vi "Begin.vi"(8 "error in":errorcluster) -> (0 "error out":errorcluster)   [LabVIEW 2018]
doc: "Called before other user functions, this VI can be used to open I/O refnums, load in file data, and do general program initialization. Notice that the <B>error out</B> terminal is simply used for data flow. Wiring it to other structures or subVIs ensures that this VI runs first."
uses:
  <vilib>/Rock Robotics/WPI/DriverStation/WPI_DriverStationRobotMode2.ctl
  <vilib>/Rock Robotics/WPI/Joystick/WPI_JoystickDeviceEnum.ctl
  <vilib>/Rock Robotics/WPI/SafetyOutput/WPI_SafetyOutputConfigMenu.ctl
  <vilib>/Rock Robotics/WPI/Solenoid/WPI_SolenoidChannel.ctl
  <vilib>/Rock Robotics/WPI/Solenoid/WPI_SolenoidValue.ctl
  <vilib>/Rock Robotics/SystemInterfaces/DIO/FPGA_DIOPWMChannel.ctl
  Robot Global Data.vi
  <vilib>/Rock Robotics/WPI/RobotDrive/WPI_RobotDriveOpen4MotorWithExistingMotors.vi
  <vilib>/Rock Robotics/WPI/RobotDrive/WPI_RobotDriveOpen2MotorWithExistingMotors.vi
  <vilib>/Rock Robotics/WPI/Solenoid/WPI_SolenoidOpenDouble.vi
  <vilib>/Rock Robotics/WPI/Solenoid/WPI_SolenoidSetEnum.vi
  <vilib>/Rock Robotics/WPI/MotorControl/WPI_MotorControlOpen SPARK.vi
panel:
  in  "Power Distribution Panel (0)":u8
  in  "Clear Sticky Faults":bool=TRUE
  out "Current Faults":bool[](array[boolean])
  out "Battery Voltage Fault":bool
  out "Temperature Fault":bool
  out "Hardware Fault":bool
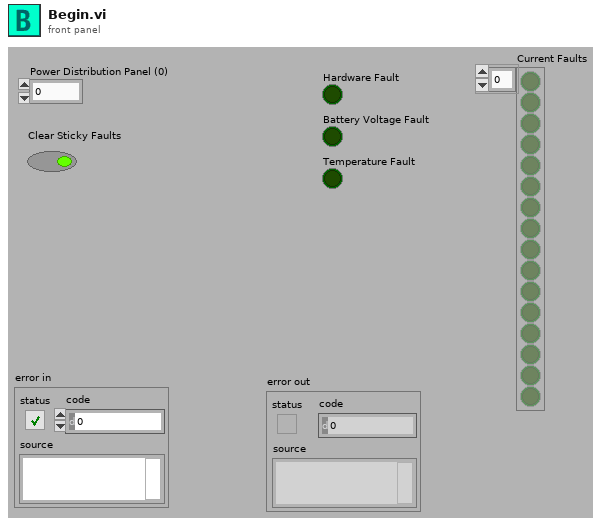
[diagram p1: front panel]
types:
  T1 = typedef "FPGA_DIOPWMChannel.ctl" = enum8{"PWM 0", "PWM 1", "PWM 2", "PWM 3", "PWM 4", "PWM 5", "PWM 6", "PWM 7", "PWM 8", "PWM 9", "PWM MXP 0", "PWM MXP 1", "PWM MXP 2", "PWM MXP 3", "PWM MXP 4", "PWM MXP 5", "PWM MXP 6", "PWM MXP 7", "PWM MXP 8", "PWM MXP 9", "Invalid"}
  T2 = typedef "WPI_SafetyOutputConfigMenu.ctl" = enum16{"Enable", "Disable"}
  T3 = typedef "WPI_SolenoidValue.ctl" = enum16{"Off", "On", "Forward", "Reverse"}
  T4 = typedef "WPI_SolenoidChannel.ctl" = enum8{"Solenoid 0", "Solenoid 1", "Solenoid 2", "Solenoid 3", "Solenoid 4", "Solenoid 5", "Solenoid 6", "Solenoid 7", "Invalid"}
  T5 = typedef "WPI_JoystickDeviceEnum.ctl" = enum16{"USB 0", "USB 1", "USB 2", "USB 3", "USB 4", "USB 5"}
  T6 = typedef "WPI_DriverStationRobotMode2.ctl" = enum16{"Autonomous Disabled", "Autonomous Enabled", "Teleop Disabled", "Teleop Enabled", "Disconnected", "Finish", "Test Disabled", "Test Enabled", "Emergency Stopped"}
  T7 = typedef "WPI_SolenoidDevRef.ctl" = cluster{"DevStatus":errorcluster, "Pneumatics Control Module":u8, "Forward Solenoid Channel":T4, "Reverse Solenoid Channel":T4}
  T8 = typedef "WPI_JoystickDevRef.ctl" = cluster{"Device":T5}
  T9 = typedef "WPI_MotorControlDeviceRef.ctl" = cluster{"DeviceStatus":errorcluster, "Type":T10, "PWM":cluster{"PWM Channel":T1, "DeadBand":T11}, "CAN":cluster{"Device Number":u8, "SetOutput VI Ref":variant, "GetOutput VI Ref":variant, "Enable VI Ref":variant, "Disable VI Ref":variant, "Data":variant}, "Invert":bool, "DIO PWM":cluster{"PWM \"Enable\" Channel":T1, "DIOChannel":T12, "PWM Rate":dbl}}
  T10 = typedef "WPI_MotorControlType.ctl" = enum16{"PWM", "CAN", "DIO PWM"}
  T11 = typedef "WPI_PWMDeadband.ctl" = cluster{"Name":string, "maxPositivePwm":i32, "minPositivePwm":i32, "centerPwm":i32, "maxNegativePwm":i32, "minNegativePwm":i32, "angularRange":u16}
  T12 = typedef "FPGA_DIOChannel.ctl" = enum8{"DIO 0", "DIO 1", "DIO 2", "DIO 3", "DIO 4", "DIO 5", "DIO 6", "DIO 7", "DIO 8", "DIO 9", "DIO MXP 0", "DIO MXP 1", "DIO MXP 2", "DIO MXP 3", "DIO MXP 4", "DIO MXP 5", "DIO MXP 6", "DIO MXP 7", "DIO MXP 8", "DIO MXP 9", "DIO MXP 10", "DIO MXP 11", "DIO MXP 12", "DIO MXP 13", "DIO MXP 14", "DIO MXP 15", "SPI Port CS1", "SPI Port CS2", "SPI Port CS3", "SPI Port MISO", "SPI Port MOSI", "Invalid"}
  T13 = typedef "WPI_RobotDriveDevRef.ctl" = cluster{"DevStatus":errorcluster, "Motors[]":T9[], "Square Inputs":bool, "Max Output":dbl}
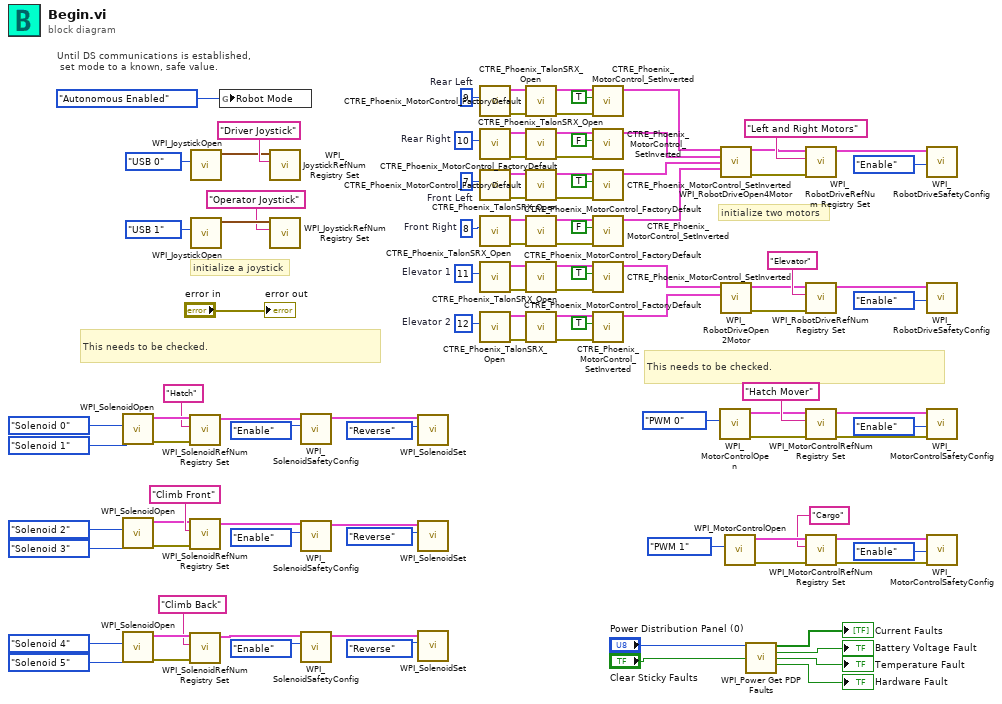
[diagram p0: block diagram]
diagram:
  w71 = u8 11  # Elevator 1
  w64 = u8 12  # Elevator 2
  w38 = u8 8  # Front Right
  w39 = u8 7  # Front Left
  w37 = u8 10  # Rear Right
  w36 = u8 9  # Rear Left
  # "This needs to be checked."
  # "This needs to be checked."
  # "initialize two motors"
  # "initialize a joystick"
  # "Until DS communications is established,\n set mode to a known, safe value."
  n1 = call-poly <vilib>:"WPI_SolenoidOpen.vi"("Reverse Solenoid Channel"=WPI_SolenoidChannel."Solenoid 1", "Forward Solenoid Channel"=WPI_SolenoidChannel."Solenoid 0" ("Solenoid Channel")) -> ("error out"=w3:errorcluster, "SolenoidDevRef"=w94:T7)  [unwired: 8 in]
  n2 = call-poly <vilib>:"WPI_SolenoidOpen.vi"("Reverse Solenoid Channel"=WPI_SolenoidChannel."Solenoid 3", "Forward Solenoid Channel"=WPI_SolenoidChannel."Solenoid 2" ("Solenoid Channel")) -> ("error out"=w2:errorcluster, "SolenoidDevRef"=w91:T7)  [unwired: 8 in]
  n3 = call-poly <vilib>:"WPI_SolenoidOpen.vi"("Reverse Solenoid Channel"=WPI_SolenoidChannel."Solenoid 5", "Forward Solenoid Channel"=WPI_SolenoidChannel."Solenoid 4" ("Solenoid Channel")) -> ("error out"=w1:errorcluster, "SolenoidDevRef"=w23:T7)  [unwired: 8 in]
  n4 = call <vilib>:"WPI_SolenoidRefNum Registry Set.vi"("error in (no error)"=w3, "refnum name"="Hatch", "SolenoidDevRef"=w94) -> ("SolenoidDevRef"=w16:T7)  [unwired: 7 in, 1 out]
  n5 = call <vilib>:"WPI_SolenoidRefNum Registry Set.vi"("error in (no error)"=w2, "refnum name"="Climb Front", "SolenoidDevRef"=w91) -> ("SolenoidDevRef"=w14:T7)  [unwired: 7 in, 1 out]
  n6 = call <vilib>:"WPI_SolenoidRefNum Registry Set.vi"("error in (no error)"=w1, "refnum name"="Climb Back", "SolenoidDevRef"=w23) -> ("SolenoidDevRef"=w12:T7)  [unwired: 7 in, 1 out]
  n7 = call <vilib>:"WPI_JoystickOpen.vi"("JoystickDevice"=WPI_JoystickDeviceEnum."USB 0") -> ("JoystickDevRef"=w29:T8)  [unwired: 10 in]
  n8 = call <vilib>:"WPI_JoystickOpen.vi"("JoystickDevice"=WPI_JoystickDeviceEnum."USB 1") -> ("JoystickDevRef"=w26:T8)  [unwired: 10 in]
  n9 = global write "Robot Global Data.vi" "Robot Mode"(WPI_DriverStationRobotMode2."Autonomous Enabled" ("Robot Mode")) -> ()
  n10 = call <vilib>:"WPI_JoystickRefNum Registry Set.vi"("refnum name"="Driver Joystick", "JoystickDevRef"=w29) -> ()  [unwired: 8 in, 2 out]
  n11 = call <vilib>:"WPI_JoystickRefNum Registry Set.vi"("refnum name"="Operator Joystick", "JoystickDevRef"=w26) -> ()  [unwired: 8 in, 2 out]
  n12 = call <vilib>:"WPI_SolenoidSafetyConfig.vi"("mode"=WPI_SafetyOutputConfigMenu."Enable", "SolenoidDevRef"=w16) -> ("SolenoidDevRef"=w15:T7)  [unwired: 8 in, 1 out]
  n13 = call <vilib>:"WPI_SolenoidSafetyConfig.vi"("mode"=WPI_SafetyOutputConfigMenu."Enable", "SolenoidDevRef"=w14) -> ("SolenoidDevRef"=w13:T7)  [unwired: 8 in, 1 out]
  n14 = call <vilib>:"WPI_SolenoidSafetyConfig.vi"("mode"=WPI_SafetyOutputConfigMenu."Enable", "SolenoidDevRef"=w12) -> ("SolenoidDevRef"=w11:T7)  [unwired: 8 in, 1 out]
  n15 = call-poly <vilib>:"WPI_SolenoidSet.vi"("Value"=WPI_SolenoidValue."Reverse", "SolenoidDevRef"=w15) -> ()  [unwired: 8 in, 2 out]
  n16 = call-poly <vilib>:"WPI_SolenoidSet.vi"("Value"=WPI_SolenoidValue."Reverse", "SolenoidDevRef"=w13) -> ()  [unwired: 8 in, 2 out]
  n17 = call-poly <vilib>:"WPI_SolenoidSet.vi"("Value"=WPI_SolenoidValue."Reverse", "SolenoidDevRef"=w11) -> ()  [unwired: 8 in, 2 out]
  n18 = call <vilib>:"CTRE_Phoenix_TalonSRX_Open.vi"("Device Number"=w36) -> ("error out"=w48:errorcluster, "CAN Talon SRX Ref"=w49:T9)  [unwired: 9 in]
  n19 = call <vilib>:"CTRE_Phoenix_TalonSRX_Open.vi"("Device Number"=w37) -> ("error out"=w50:errorcluster, "CAN Talon SRX Ref"=w51:T9)  [unwired: 9 in]
  n20 = call <vilib>:"CTRE_Phoenix_TalonSRX_Open.vi"("Device Number"=w39) -> ("error out"=w52:errorcluster, "CAN Talon SRX Ref"=w53:T9)  [unwired: 9 in]
  n21 = call <vilib>:"CTRE_Phoenix_TalonSRX_Open.vi"("Device Number"=w38) -> ("error out"=w54:errorcluster, "CAN Talon SRX Ref"=w55:T9)  [unwired: 9 in]
  n22 = call <vilib>:"CTRE_Phoenix_TalonSRX_Open.vi"("Device Number"=w71) -> ("error out"=w7:errorcluster, "CAN Talon SRX Ref"=w69:T9)  [unwired: 9 in]
  n23 = call <vilib>:"CTRE_Phoenix_TalonSRX_Open.vi"("Device Number"=w64) -> ("error out"=w5:errorcluster, "CAN Talon SRX Ref"=w66:T9)  [unwired: 9 in]
  n24 = call <vilib>:"CTRE_Phoenix_MotorControl_FactoryDefault.vi"("error in"=w48, "PhoenixMotorControlDevRef"=w49) -> ("error out"=w57:errorcluster, "PhoenixMotorControlDevRef"=w56:T9)  [unwired: 8 in]
  n25 = call <vilib>:"CTRE_Phoenix_MotorControl_FactoryDefault.vi"("error in"=w50, "PhoenixMotorControlDevRef"=w51) -> ("error out"=w59:errorcluster, "PhoenixMotorControlDevRef"=w58:T9)  [unwired: 8 in]
  n26 = call <vilib>:"CTRE_Phoenix_MotorControl_FactoryDefault.vi"("error in"=w52, "PhoenixMotorControlDevRef"=w53) -> ("error out"=w61:errorcluster, "PhoenixMotorControlDevRef"=w60:T9)  [unwired: 8 in]
  n27 = call <vilib>:"CTRE_Phoenix_MotorControl_FactoryDefault.vi"("error in"=w54, "PhoenixMotorControlDevRef"=w55) -> ("error out"=w63:errorcluster, "PhoenixMotorControlDevRef"=w62:T9)  [unwired: 8 in]
  n28 = call <vilib>:"CTRE_Phoenix_MotorControl_FactoryDefault.vi"("error in"=w7, "PhoenixMotorControlDevRef"=w69) -> ("error out"=w6:errorcluster, "PhoenixMotorControlDevRef"=w68:T9)  [unwired: 8 in]
  n29 = call <vilib>:"CTRE_Phoenix_MotorControl_FactoryDefault.vi"("error in"=w5, "PhoenixMotorControlDevRef"=w66) -> ("error out"=w4:errorcluster, "PhoenixMotorControlDevRef"=w67:T9)  [unwired: 8 in]
  n30 = call <vilib>:"CTRE_Phoenix_MotorControl_SetInverted.vi"("error in (no error)"=w57, "Invert?"=TRUE, "PhoenixMotorControlDevRef"=w56) -> ("PhoenixMotorControlDevRef"=w47:T9)  [unwired: 7 in, 1 out]
  n31 = call <vilib>:"CTRE_Phoenix_MotorControl_SetInverted.vi"("error in (no error)"=w59, "Invert?"=FALSE, "PhoenixMotorControlDevRef"=w58) -> ("PhoenixMotorControlDevRef"=w42:T9)  [unwired: 7 in, 1 out]
  n32 = call <vilib>:"CTRE_Phoenix_MotorControl_SetInverted.vi"("error in (no error)"=w61, "Invert?"=TRUE, "PhoenixMotorControlDevRef"=w60) -> ("PhoenixMotorControlDevRef"=w45:T9)  [unwired: 7 in, 1 out]
  n33 = call <vilib>:"CTRE_Phoenix_MotorControl_SetInverted.vi"("error in (no error)"=w63, "Invert?"=FALSE, "PhoenixMotorControlDevRef"=w62) -> ("PhoenixMotorControlDevRef"=w40:T9)  [unwired: 7 in, 1 out]
  n34 = call <vilib>:"CTRE_Phoenix_MotorControl_SetInverted.vi"("error in (no error)"=w6, "Invert?"=TRUE, "PhoenixMotorControlDevRef"=w68) -> ("PhoenixMotorControlDevRef"=w84:T9)  [unwired: 7 in, 1 out]
  n35 = call <vilib>:"CTRE_Phoenix_MotorControl_SetInverted.vi"("error in (no error)"=w4, "Invert?"=TRUE, "PhoenixMotorControlDevRef"=w67) -> ("PhoenixMotorControlDevRef"=w85:T9)  [unwired: 7 in, 1 out]
  n36 = call-poly <vilib>:"WPI_MotorControlOpen.vi"("PWM Channel"=FPGA_DIOPWMChannel."PWM 0") -> ("error out"=w72:errorcluster, "MotorControlDeviceRef"=w73:T9)  [unwired: 9 in]
  n37 = call-poly <vilib>:"WPI_RobotDriveOpen4Motor.vi"("Rear Left Motor Dev Ref"=w47, "Rear Right Motor Dev Ref"=w42, "Front Left Motor Dev Ref"=w45, "Front Right Motor Dev Ref"=w40) -> ("RobotDriveDevRef"=w31:T13, "error out"=w33:errorcluster)  [unwired: 10 in]
  n38 = call-poly <vilib>:"WPI_RobotDriveOpen2Motor.vi"("Right Motor Dev Ref"=w85, "Left Motor Dev Ref"=w84) -> ("error out"=w8:errorcluster, "RobotDriveDevRef"=w88:T13)  [unwired: 8 in]
  n39 = call-poly <vilib>:"WPI_MotorControlOpen.vi"("PWM Channel"=FPGA_DIOPWMChannel."PWM 1") -> ("error out"=w83:errorcluster, "MotorControlDeviceRef"=w82:T9)  [unwired: 9 in]
  n40 = call <vilib>:"WPI_Power Get PDP Faults.vi"("Power Distribution Panel (0)"="Power Distribution Panel (0)", "Clear Sticky Faults"="Clear Sticky Faults") -> ("Current Faults"=→"Current Faults":bool[], "Battery Voltage Fault"=→"Battery Voltage Fault":bool, "Temperature Fault"=→"Temperature Fault":bool, "Hardware Fault"=→"Hardware Fault":bool)  [unwired: 9 in, 1 out]
  n41 = call <vilib>:"WPI_RobotDriveRefNum Registry Set.vi"("error in (no error)"=w33, "refnum name"="Left and Right Motors", "RobotDriveDevRef"=w31) -> ("RobotDriveDevRef"=w34:T13)  [unwired: 1 in, 7 out]
  n42 = call <vilib>:"WPI_RobotDriveRefNum Registry Set.vi"("error in (no error)"=w8, "refnum name"="Elevator", "RobotDriveDevRef"=w88) -> ("RobotDriveDevRef"=w87:T13)  [unwired: 1 in, 7 out]
  n43 = call <vilib>:"WPI_MotorControlRefNum Registry Set.vi"("error in (no error)"=w72, "refnum name"="Hatch Mover", "MotorControlDevRef"=w73) -> ("error out"=w74:errorcluster, "MotorControlDevRef"=w75:T9)  [unwired: 7 in]
  n44 = call <vilib>:"WPI_MotorControlRefNum Registry Set.vi"("error in (no error)"=w83, "refnum name"="Cargo", "MotorControlDevRef"=w82) -> ("error out"=w81:errorcluster, "MotorControlDevRef"=w80:T9)  [unwired: 7 in]
  n45 = call <vilib>:"WPI_RobotDriveSafetyConfig.vi"("mode"=WPI_SafetyOutputConfigMenu."Enable", "RobotDriveDevRef"=w34) -> ()  [unwired: 8 in, 2 out]
  n46 = call <vilib>:"WPI_RobotDriveSafetyConfig.vi"("mode"=WPI_SafetyOutputConfigMenu."Enable", "RobotDriveDevRef"=w87) -> ()  [unwired: 8 in, 2 out]
  n47 = call <vilib>:"WPI_MotorControlSafetyConfig.vi"("error in (no error)"=w74, "mode"=WPI_SafetyOutputConfigMenu."Enable", "MotorControlDevRef"=w75) -> ()  [unwired: 7 in, 2 out]
  n48 = call <vilib>:"WPI_MotorControlSafetyConfig.vi"("error in (no error)"=w81, "mode"=WPI_SafetyOutputConfigMenu."Enable", "MotorControlDevRef"=w80) -> ()  [unwired: 7 in, 2 out]
  "error out" <- "error in"
